vi "Optimize RF Power.vi"(4 "MC Error in":errorcluster, 5 "Lock-in Error In":errorcluster, 6 "Time to read at power [ms]":i32=500, 8 "Spectral Data In":T2={"PDT Amp [v]"=0.0, "RIS Amp [v]"=0.0, "B-Field"=[], "All In-Phase Scan Spectra"=[], "Model Select"=enum."OneCompRISTwoPDT", "Fit Each Scan"=FALSE, "PDT Center [g]"=0.0, "In-Phase Average Spectra"=[], "In-Phase Median Spectra"=[], "Out-Phase Median Spectra"=[], "Out-Phase Average Spectra"=[], "Fit Spectra"=[], "Fit No-Baseline Spectra"=[], "All Out-Phase Scan Spectra"=[], "Baseline Offset Correction"=FALSE, "In-Phase Offset [v]"=0.0, "Out-Phase Offset [v]"=0.0, "Ch2 Input\n(Balance)"=[], "Ch3 Input\n(Phase)"=[], "Ch4 Input\n(AFC)"=[], "Fit Pars"=[], "Fit Pars Errors"=[], "Fit Pars Labels"=[], "Raw Scan DAQ Data"=[], "Bad Scans Indicies"=[], "Good In-Phase Scan Spectra"=[], "Good Out-Phase Scan Spectra"=[], "Bad In-Phase Scan Spectra"=[], "Bad Out-Phase Scan Spectra"=[], "Number of bad scans"=0, "Fit History"=[], "PDT Amp. History/Set [v]"=[], "RIS Amp. History/Set [v]"=[], "RIS Amp. History/Scan [v]"=[], "All Shifted B-Fields"=[], "Good Shifted B-Fields"=[], "Ch5 Input\n(SpO2)"=[], "Ch6 Input\n(BPM)"=[], "Global SNR"=0.0, "Fit Error History"=[], "SNR History"=[]} {"Global SNR" min=0.0; "PDT Center [g]" min=0.0; "RIS Amp [v]" min=0.0; "PDT Amp [v]" min=0.0}, 9 "Hardware Parameters In":T1={"Scan Calibration [G/V]"=0.0, "Modulation Calibration [G/V]"=0.0, "Modulation Phase [deg]"=0.0, "Modulation Frequency [Hz]"=0.0, "Attenuation [dB]"=0, "Input Channel Count"=0, "Time constant"=7, "Sensitivity"=17, "Frequency Output Voltage [V]"=0.0, "Phase Output Voltage [V]"=0.0, "Lock-in Offset Compensation"=FALSE, "RF [GHz]"=0.0, "Q Start"=0.0, "Q End"=0.0, "Balance"=0.0, "Phase Error"=0.0, "AFC Error"=0.0, "AFC"=FALSE, "Magnet Rotation"=FALSE, "Balance Scaling Factor"=1.0, "Phase Error Scaling Factor"=1.0, "AFC Error Scaling Factor"=1.0, "Frequency Counter ID"="", "Sweep Waveform"=enum."Sawtooth", "Q-Factor Scale"=0.0, " Q-Data Scale"=0.0, " Q-Data Offset"=0.0, "Magnet Rotation Slope"=0.0, "Magnet Rotation Offset"=0.0, "Phase Sweep Resolution"=0.0, "Hardware Version Number"="", "Spectrometer ID Number"=0, "Spectrometer Name"="", "Lock in Saturation"=0.0, "Balance Threshold"=0.0, "Phase Error Threshold"=0.0, "AFC Error Threshold"=0.0, "Linear Actuator Length"=0.0, "Lock-in OK?"=FALSE, "Ignore Lock-in Comm. Failure"=FALSE, "Gradient Addresses"=[], "Gradient Calibrations [G/A*mm]"=[], "Gradient Power Supplies"=[], "Lock-in Address"="", "Magnet Type"=enum."RRI", "Camera Names"=[], "Sweep Limit [Gauss]"=0.0, "Modulation Limit [Gauss]"=0.0, "Balance Threshold Exceeded?"=FALSE, "Phase Threshold Exceeded?"=FALSE, "AFC Threshold Exceeded?"=FALSE, "Consecutive Re-tune attempts"=0, "Reverse Sweep Slope [sec]"=0.0, "Reverse Sweep Offset [G]"=0.0, "AFC Field Correction [V/MHz]"=0.0, "Active Gradients (X Y Z)"=[], "SpO2 Calibration [SpO2/V]"=1.0, "Heart Rate Calibration [BPM/V]"=1.0, "Thermocouple Channel"=""} {"Sensitivity" items=["", "2 nV", "5 nV", "10 nV", "20 nV", "50 nV", "100 nV", "200 nV", "500 nV", "1 uV", "2 uV", "5 uV", "10 uV", "20 uV", "50 uV", "100 uV", "200 uV", "500 uV", "1 mV", "2 mV", "5 mV", "10 mV", "20 mV", "50 mV", "100 mV", "200 mV", "500 mV", "1 V"]; "Time constant" items=["10 us", "20 us", "40 us", "80 us", "160 us", "320 us", "640 us", "5 ms", "10 ms", "20 ms", "50 ms", "100 ms", "200 ms", "500 ms", "1 s", "2 s", "5 s", "10 s", "20 s", "50 s", "100 s", "200 s", "500 s", "1 ks", "2 ks", "5 ks", "10 ks", "20 ks", "50 ks", "100 ks"]}) -> (0 "Resultant Attenuation [dB]":u16, 1 "MC error out":errorcluster, 2 "Lock-in error out":errorcluster, 3 "Hardware Parameters Out":T1={"Scan Calibration [G/V]"=0.0, "Modulation Calibration [G/V]"=0.0, "Modulation Phase [deg]"=0.0, "Modulation Frequency [Hz]"=0.0, "Attenuation [dB]"=0, "Input Channel Count"=0, "Time constant"=7, "Sensitivity"=17, "Frequency Output Voltage [V]"=0.0, "Phase Output Voltage [V]"=0.0, "Lock-in Offset Compensation"=FALSE, "RF [GHz]"=0.0, "Q Start"=0.0, "Q End"=0.0, "Balance"=0.0, "Phase Error"=0.0, "AFC Error"=0.0, "AFC"=FALSE, "Magnet Rotation"=FALSE, "Balance Scaling Factor"=1.0, "Phase Error Scaling Factor"=1.0, "AFC Error Scaling Factor"=1.0, "Frequency Counter ID"="", "Sweep Waveform"=enum."Sawtooth", "Q-Factor Scale"=0.0, " Q-Data Scale"=0.0, " Q-Data Offset"=0.0, "Magnet Rotation Slope"=0.0, "Magnet Rotation Offset"=0.0, "Phase Sweep Resolution"=0.0, "Hardware Version Number"="", "Spectrometer ID Number"=0, "Spectrometer Name"="", "Lock in Saturation"=0.0, "Balance Threshold"=0.0, "Phase Error Threshold"=0.0, "AFC Error Threshold"=0.0, "Linear Actuator Length"=0.0, "Lock-in OK?"=FALSE, "Ignore Lock-in Comm. Failure"=FALSE, "Gradient Addresses"=[], "Gradient Calibrations [G/A*mm]"=[], "Gradient Power Supplies"=[], "Lock-in Address"="", "Magnet Type"=enum."RRI", "Camera Names"=[], "Sweep Limit [Gauss]"=0.0, "Modulation Limit [Gauss]"=0.0, "Balance Threshold Exceeded?"=FALSE, "Phase Threshold Exceeded?"=FALSE, "AFC Threshold Exceeded?"=FALSE, "Consecutive Re-tune attempts"=0, "Reverse Sweep Slope [sec]"=0.0, "Reverse Sweep Offset [G]"=0.0, "AFC Field Correction [V/MHz]"=0.0, "Active Gradients (X Y Z)"=[], "SpO2 Calibration [SpO2/V]"=1.0, "Heart Rate Calibration [BPM/V]"=1.0, "Thermocouple Channel"=""} {"Sensitivity" items=["", "2 nV", "5 nV", "10 nV", "20 nV", "50 nV", "100 nV", "200 nV", "500 nV", "1 uV", "2 uV", "5 uV", "10 uV", "20 uV", "50 uV", "100 uV", "200 uV", "500 uV", "1 mV", "2 mV", "5 mV", "10 mV", "20 mV", "50 mV", "100 mV", "200 mV", "500 mV", "1 V"]; "Time constant" items=["10 us", "20 us", "40 us", "80 us", "160 us", "320 us", "640 us", "5 ms", "10 ms", "20 ms", "50 ms", "100 ms", "200 ms", "500 ms", "1 s", "2 s", "5 s", "10 s", "20 s", "50 s", "100 s", "200 s", "500 s", "1 ks", "2 ks", "5 ks", "10 ks", "20 ks", "50 ks", "100 ks"]})   [LabVIEW 2016]
uses:
  Types/Hardware Parameters.ctl
  Types/Spectral Data.ctl
  Types/Fitting Model Selection.ctl
  <vilib>/Analysis/NI_AALBase.lvlib
panel:
  out "Max Attenuation Reached":bool
  out "Live Data at Power":dbl[](graph)
  out "Power Points":dbl[](array[numeric])
  out "Amplitude vs. Attenuation Steps (3db/step)":dbl[](graph)
  out "Optimized Attenuation [dB]":u16 max=31 step=1
  out "Current Attenuation [dB]":u16 max=31 step=1
  in  "Cases":T4(ring)
  # "Bridge I/O"
  # "Magnet Rotation"
  # "Field Calibration"
  # "Lock In Amplifier"
  # "Spectrometer Information"
  # "DAQ Settings"
  # "Gradient Coils and Field"
  # "X"
  # "Y"
  # "Z"
  # "Q-Measurements"
  # "Bridge I/O"
  # "Magnet Rotation"
  # "Field Calibration"
  # "Lock In Amplifier"
  # "Spectrometer Information"
  # "DAQ Settings"
  # "Gradient Coils and Field"
  # "X"
  # "Y"
  # "Z"
  # "Q-Measurements"
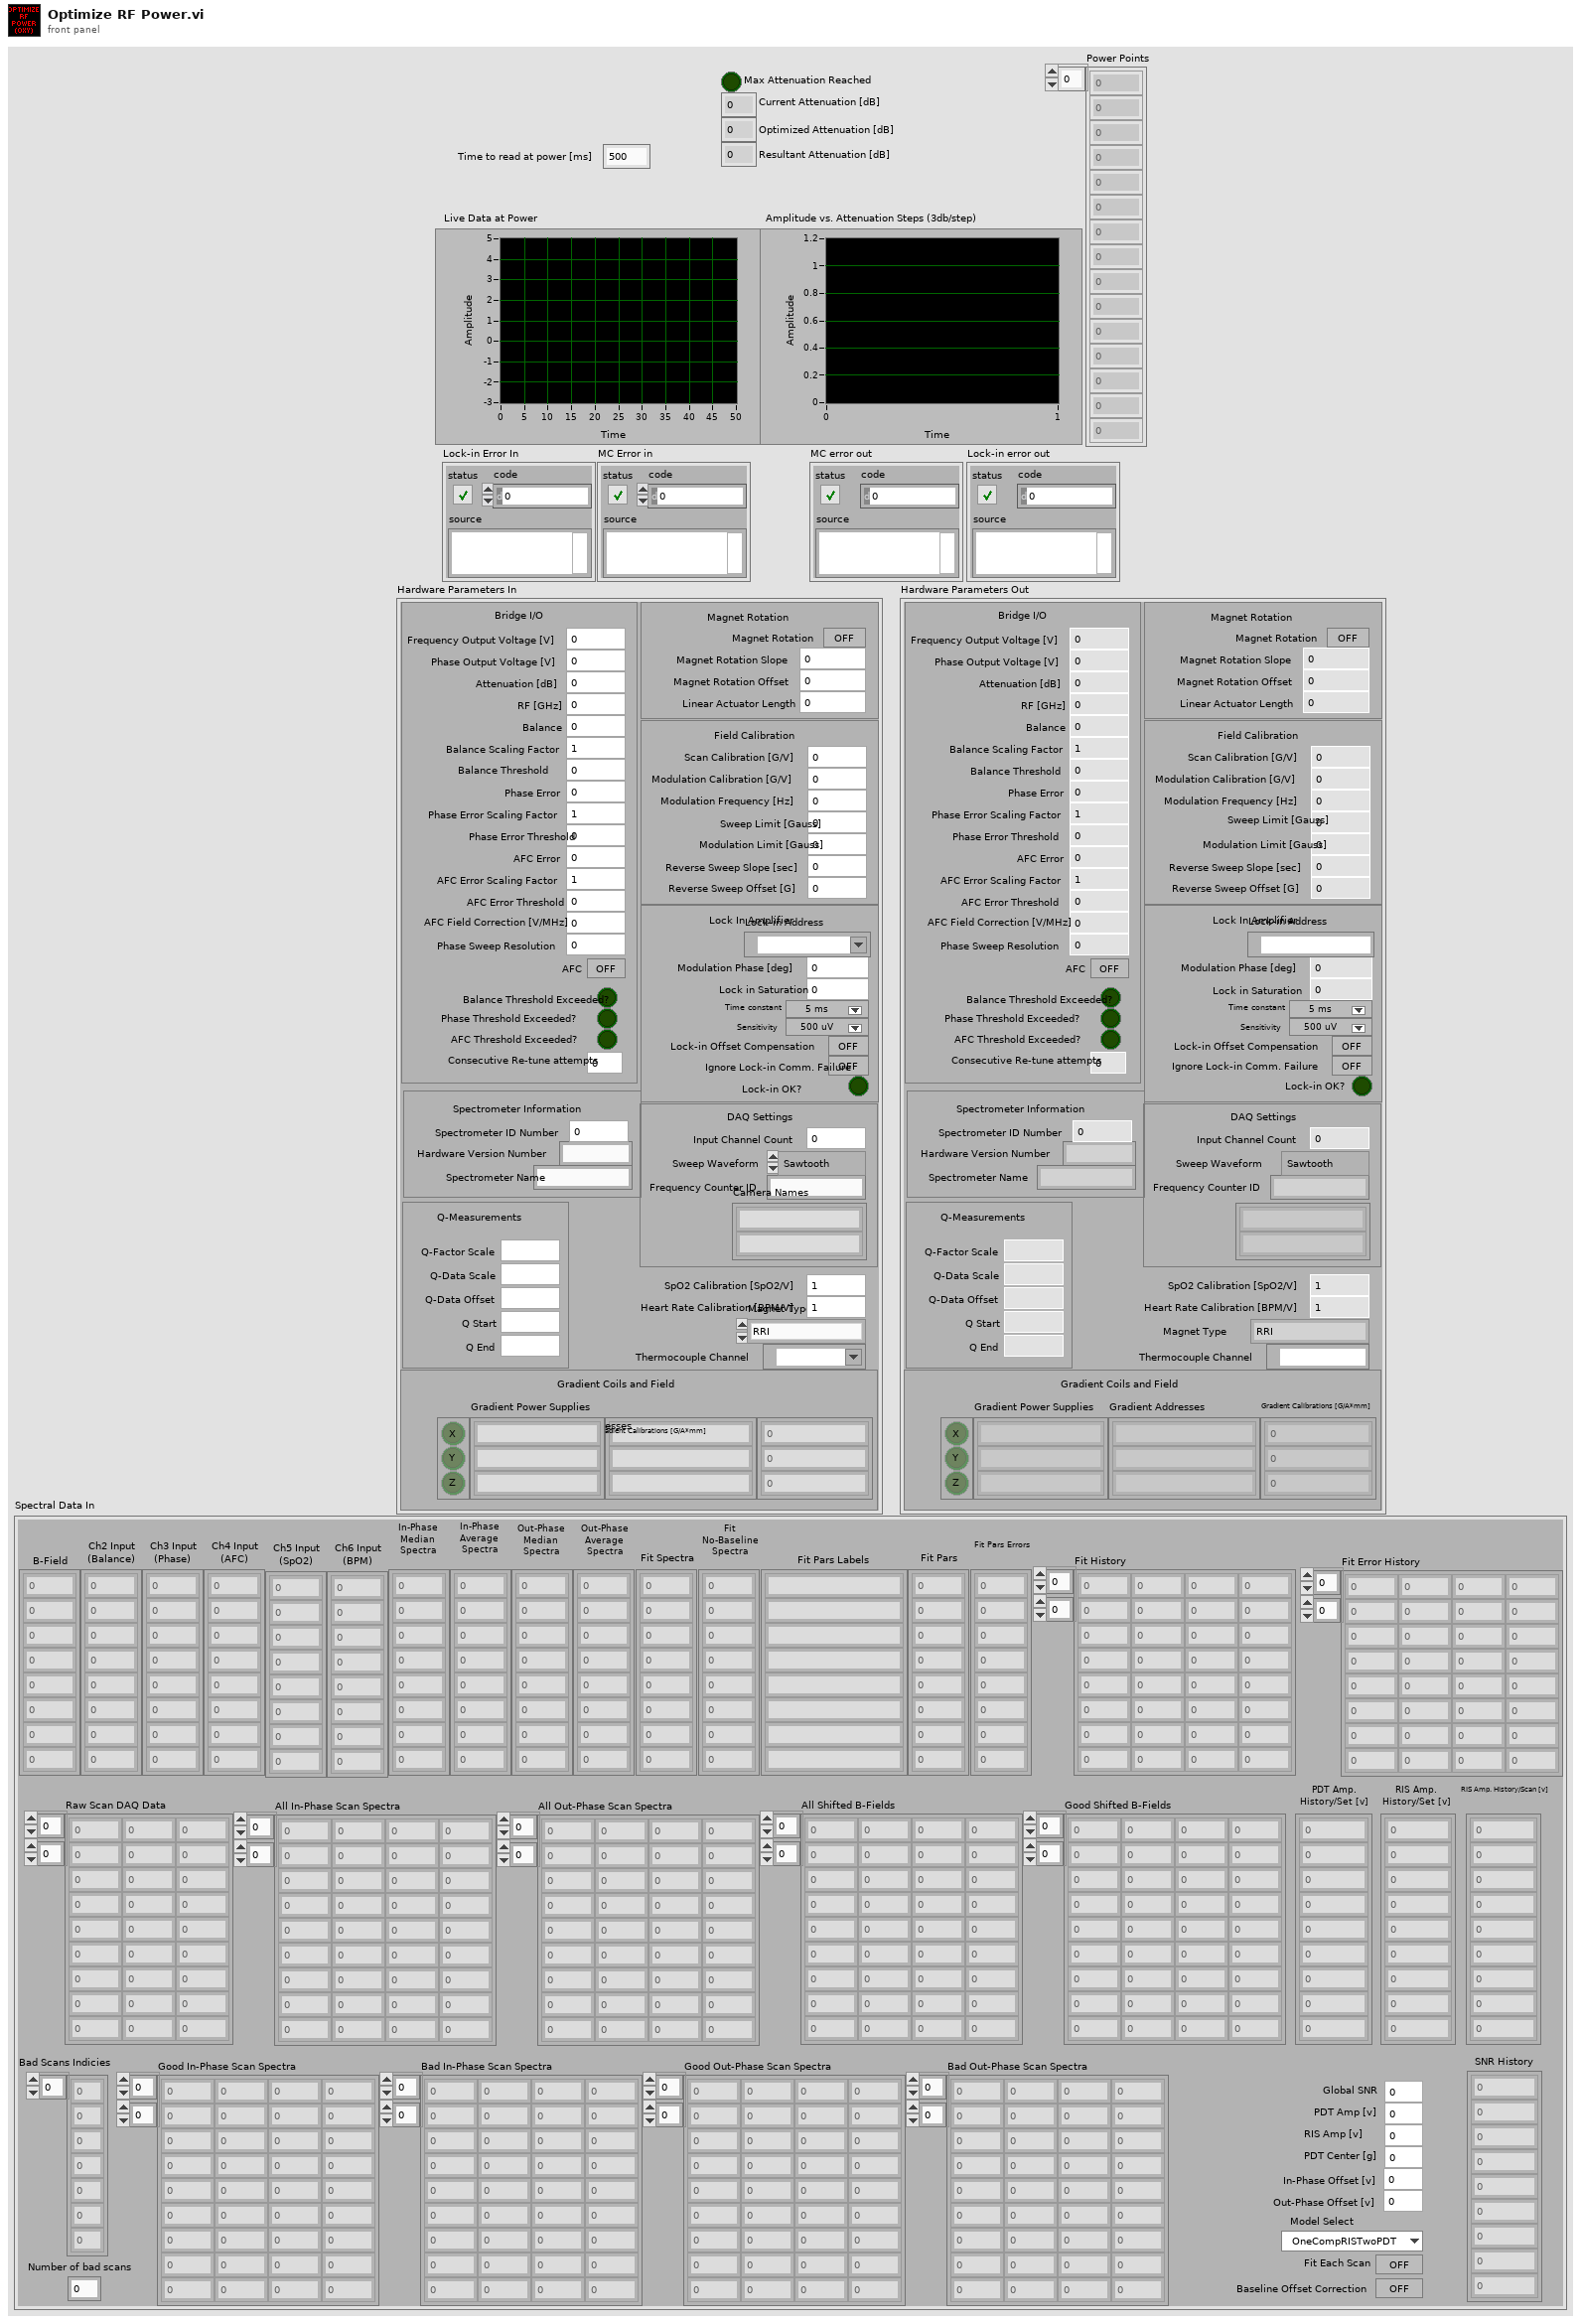
[diagram p1: front panel]
types:
  T1 = typedef "Hardware Parameters.ctl" = cluster{"Scan Calibration [G/V]":dbl, "Modulation Calibration [G/V]":dbl, "Modulation Phase [deg]":dbl, "Modulation Frequency [Hz]":dbl, "Attenuation [dB]":u16, "Input Channel Count":i32, "Time constant":u16, "Sensitivity":u16, "Frequency Output Voltage [V]":dbl, "Phase Output Voltage [V]":dbl, "Lock-in Offset Compensation":bool, "RF [GHz]":dbl, "Q Start":dbl, "Q End":dbl, "Balance":dbl, "Phase Error":dbl, "AFC Error":dbl, "AFC":bool, "Magnet Rotation":bool, "Balance Scaling Factor":dbl, "Phase Error Scaling Factor":dbl, "AFC Error Scaling Factor":dbl, "Frequency Counter ID":string, "Sweep Waveform":enum16{"Sine Wave", "Square Wave", "Sawtooth", "Triangle Wave"}, "Q-Factor Scale":dbl, " Q-Data Scale":dbl, " Q-Data Offset":dbl, "Magnet Rotation Slope":dbl, "Magnet Rotation Offset":dbl, "Phase Sweep Resolution":dbl, "Hardware Version Number":string, "Spectrometer ID Number":i32, "Spectrometer Name":string, "Lock in Saturation":dbl, "Balance Threshold":dbl, "Phase Error Threshold":dbl, "AFC Error Threshold":dbl, "Linear Actuator Length":dbl, "Lock-in OK?":bool, "Ignore Lock-in Comm. Failure":bool, "Gradient Addresses":string[], "Gradient Calibrations [G/A*mm]":dbl[], "Gradient Power Supplies":string[], "Lock-in Address":refnum<visa-resource-name>, "Magnet Type":enum16{"RRI", "BARDA", "Whole Body Permanent", "RRI Electromagnet"}, "Camera Names":string[], "Sweep Limit [Gauss]":dbl, "Modulation Limit [Gauss]":dbl, "Balance Threshold Exceeded?":bool, "Phase Threshold Exceeded?":bool, "AFC Threshold Exceeded?":bool, "Consecutive Re-tune attempts":i32, "Reverse Sweep Slope [sec]":dbl, "Reverse Sweep Offset [G]":dbl, "AFC Field Correction [V/MHz]":dbl, "Active Gradients (X Y Z)":bool[], "SpO2 Calibration [SpO2/V]":dbl, "Heart Rate Calibration [BPM/V]":dbl, "Thermocouple Channel":tag}
  T2 = typedef "Spectral Data.ctl" = cluster{"PDT Amp [v]":dbl, "RIS Amp [v]":dbl, "B-Field":dbl[], "All In-Phase Scan Spectra":dbl[][], "Model Select":T3, "Fit Each Scan":bool, "PDT Center [g]":dbl, "In-Phase Average Spectra":dbl[], "In-Phase Median Spectra":dbl[], "Out-Phase Median Spectra":dbl[], "Out-Phase Average Spectra":dbl[], "Fit Spectra":dbl[], "Fit No-Baseline Spectra":dbl[], "All Out-Phase Scan Spectra":dbl[][], "Baseline Offset Correction":bool, "In-Phase Offset [v]":dbl, "Out-Phase Offset [v]":dbl, "Ch2 Input\n(Balance)":dbl[], "Ch3 Input\n(Phase)":dbl[], "Ch4 Input\n(AFC)":dbl[], "Fit Pars":dbl[], "Fit Pars Errors":dbl[], "Fit Pars Labels":string[], "Raw Scan DAQ Data":dbl[][], "Bad Scans Indicies":i32[], "Good In-Phase Scan Spectra":dbl[][], "Good Out-Phase Scan Spectra":dbl[][], "Bad In-Phase Scan Spectra":dbl[][], "Bad Out-Phase Scan Spectra":dbl[][], "Number of bad scans":i32, "Fit History":dbl[][], "PDT Amp. History/Set [v]":dbl[], "RIS Amp. History/Set [v]":dbl[], "RIS Amp. History/Scan [v]":dbl[], "All Shifted B-Fields":dbl[][], "Good Shifted B-Fields":dbl[][], "Ch5 Input\n(SpO2)":dbl[], "Ch6 Input\n(BPM)":dbl[], "Global SNR":dbl, "Fit Error History":dbl[][], "SNR History":dbl[]}
  T3 = typedef "Fitting Model Selection.ctl" = enum16{"OneCompRIS", "OneCompRISTwoPDT", "OneCompRISRev", "OneCompRISTwoPDTRev", "LiPc", "TwoLiPc", "ThreeLiPc", "FourLiPc", "PDTCalibration", "CE_Ink", "Printex", "MelaninTwoPDT"}
  T4 = enum16{"Delay", "Collect Data", "Reduce Power", "Increase Power", "Compare", "Complete"}
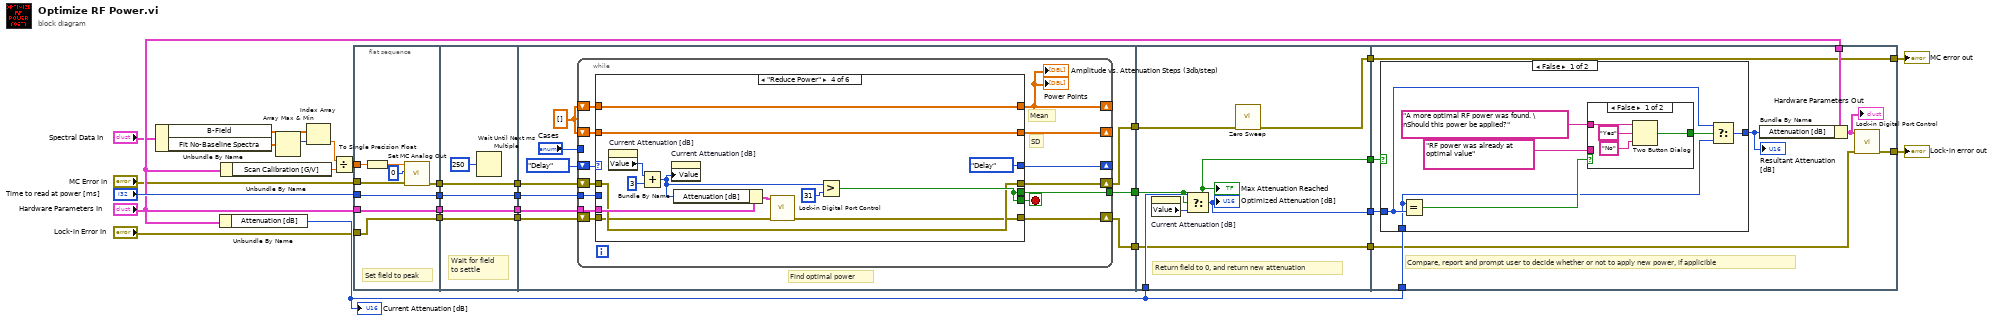
[diagram p0: block diagram]
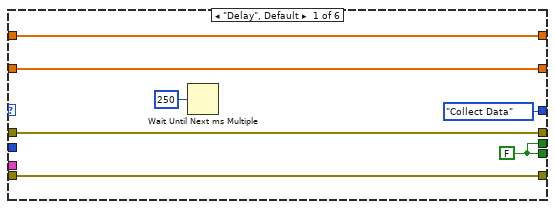
[diagram p2: hidden frame]
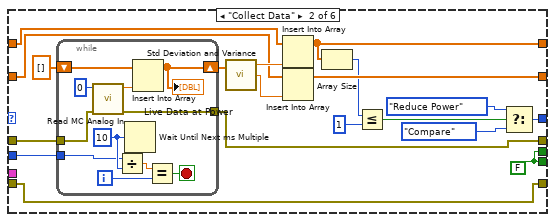
[diagram p3: hidden frame]
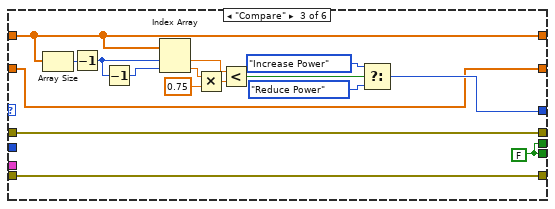
[diagram p4: hidden frame]
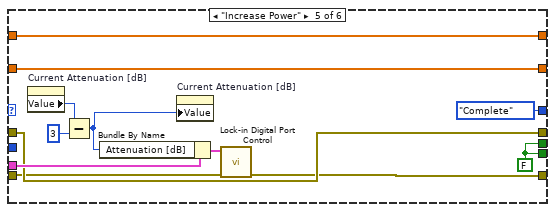
[diagram p5: hidden frame]
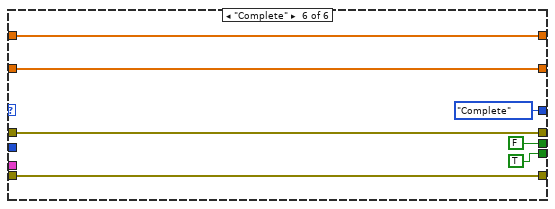
[diagram p6: hidden frame]
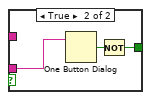
[diagram p7: hidden frame]
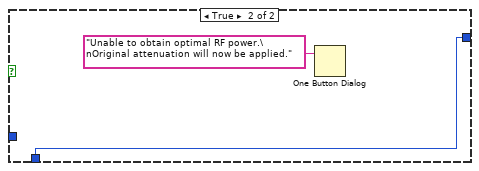
[diagram p8: hidden frame]
diagram:
  n1 = Unbundle By Name("Spectral Data In") -> ("B-Field"=w14:dbl[], "Fit No-Baseline Spectra"=w16:dbl[])
  n2 = Unbundle By Name("Hardware Parameters In") -> ("Attenuation [dB]"=w19:u16)
  "Current Attenuation [dB]" <- w19
  n3 = Unbundle By Name("Hardware Parameters In") -> ("Scan Calibration [G/V]"=w22:dbl)
  n4 = Array Max & Min(array=w16) -> (max index (indices)=w15:i32)  [unwired: 3 out]
  n5 = Index Array(array=w14, index=w15) -> (element=w13:dbl)
  n6 = Divide(x=w13, y=w22) -> (x/y=w29:dbl)
  n7 = flat-sequence {
    tunnel: w29 -> [w35]
    tunnel: "Time to read at power [ms]" -> [w37]
    tunnel: [w37] -> w28
    tunnel: "Hardware Parameters In" -> [w33]
    tunnel: [w33] -> w23
    tunnel: [w32] -> w11
    tunnel: "MC Error in" -> [w31]
    tunnel: "Lock-in Error In" -> [w30]
    tunnel: [w30] -> w7
    tunnel: [w41] -> w27
    tunnel: w28 -> [w41]
    tunnel: [w40] -> w24
    tunnel: w23 -> [w40]
    tunnel: [w39] -> w12
    tunnel: w11 -> [w39]
    tunnel: [w38] -> w8
    tunnel: w7 -> [w38]
    tunnel: w27 -> [w51]
    tunnel: [w48] -> w25
    tunnel: w24 -> [w47]
    tunnel: w12 -> [w46]
    tunnel: w8 -> [w45]
    tunnel: [w44] -> w6
    tunnel: [w43] -> w5
    tunnel: w25 -> [w155]
    tunnel: w19 -> [w158]
    tunnel: [w156] -> w21
    tunnel: [w155] -> w20
    tunnel: w6 -> [w154]
    tunnel: w5 -> [w153]
    tunnel: [w153] -> w4
    tunnel: [w152] -> w3
    tunnel: w21 -> [w167]
    tunnel: w20 -> [w166]
    tunnel: w19 -> [w165]
    tunnel: "Hardware Parameters In" -> [w163]
    tunnel: w4 -> [w161]
    tunnel: w3 -> [w160]
    tunnel: [w160] -> w2
    tunnel: [w159] -> w1
    frame #0 {
      # "Set field to peak"
      n8 = To Single Precision Float(number=w35) -> (single precision float=w34:sgl)
      n9 = call "Set MC Analog Out.vi"("error in (no error)"=w31, "Channel"=0, "Output Voltage"=w34) -> ("error out"=w32:errorcluster)  [unwired: 8 in]
    }
    frame #1 {
      # "Wait for field \nto settle"
      n10 = Wait Until Next ms Multiple(millisecond multiple=u32 250) -> ()  [unwired: 1 out]
    }
    frame #2 {
      w49 = dbl[] []
      # "Find optimal power"
      n11 = while {
        shift-right: [w65] -> _
        shift-left: T4."Delay" ("Cases") -> [w63]
        tunnel: "Cases" -> [_]
        tunnel: w51 -> [w64]
        shift-right: [w59] -> _
        shift-left: w49 -> [w62]
        shift-right: [w61] -> _
        shift-left: w49 -> [w60]
        tunnel: [w58] -> w48
        tunnel: w47 -> [w57]
        shift-right: [w55] -> w44
        shift-left: w46 -> [w56]
        shift-right: [w54] -> w43
        shift-left: w45 -> [w53]
        stop <- w66 stop-if-true
        # "SD"
        # "Mean"
        n12 = case shown="\"Reduce Power\"" w63 {
          tunnel: [w69 w77 w106 w126 w139 TRUE] -> w66
          tunnel: [T4."Collect Data" ("Cases") w80 w119 T4."Delay" ("Cases") T4."Complete" ("Cases") T4."Complete" ("Cases")] -> w65
          tunnel: w64 -> [_ w91 _ _ _ _]
          tunnel: [w71 w85 w115 w130 w142 w149] -> w59
          tunnel: w62 -> [w71 w89 w115 w130 w142 w149]
          tunnel: [w70 w87 w114 w129 w141 w148] -> w61
          tunnel: w60 -> [w70 w86 w114 w129 w141 w148]
          tunnel: [w69 w77 w106 w126 w139 FALSE] -> w58
          tunnel: w57 -> [_ _ _ w125 w136 _]
          tunnel: w56 -> [w68 w76 w105 w122 w135 w146]
          tunnel: [w68 w75 w105 w122 w135 w146] -> w55
          tunnel: [w67 w74 w104 w121 w133 w145] -> w54
          tunnel: w53 -> [w67 w74 w104 w120 w134 w145]
          frame "Delay", Default {
            w69 = FALSE
            n13 = Wait Until Next ms Multiple(millisecond multiple=u32 250) -> ()  [unwired: 1 out]
          }
          frame "Collect Data" {
            w77 = FALSE
            n14 = while {
              shift-right: [w97] -> w92
              shift-left: dbl[] [] -> [w99]
              tunnel: w91 -> [w98]
              tunnel: w76 -> [w94]
              tunnel: [w93] -> w75
              i -> [w103]
              stop <- w102 stop-if-true
              w101 = u32 10 ("millisecond multiple")
              n15 = call "Read MC Analog In.vi"("error in (no error)"=w94, "channel"=0 ("Channel")) -> ("error out"=w93:errorcluster, "Voltage Input"=w96:dbl)  [unwired: 8 in]
              n16 = Divide(x=w98, y=w101) -> (x/y=w100:dbl)
              n17 = Wait Until Next ms Multiple(millisecond multiple=w101) -> ()  [unwired: 1 out]
              n18 = Insert Into Array(array=w99, new element=w96) -> (w97:dbl[])  [unwired: 1 in]
              "Live Data at Power" <- w97
              n19 = Equal?(x=w100, y=w103) -> (x = y?=w102:bool)
            }
            n20 = call <vilib>:"Std Deviation and Variance.vi"("X"=w92) -> ("mean"=w90:dbl, "standard deviation"=w88:dbl)  [unwired: 1 in, 1 out]
            n21 = Insert Into Array(array=w89, new element=w90) -> (w85:dbl[])  [unwired: 1 in]
            n22 = Insert Into Array(array=w86, new element=w88) -> (w87:dbl[])  [unwired: 1 in]
            n23 = Array Size(array=w85) -> (size(s)=w84:i32)
            n24 = Less Or Equal?(x=w84, y=1) -> (x <= y?=w82:bool)
            n25 = Select(t=T4."Reduce Power" ("Cases"), s=w82, f=T4."Compare" ("Cases")) -> (s? t:f=w80:T4)
          }
          frame "Compare" {
            w106 = FALSE
            n26 = Array Size(array=w115) -> (size(s)=w113:i32)
            n27 = Decrement(x=w113) -> (x-1=w111:i32)
            n28 = Decrement(x=w111) -> (x-1=w112:i32)
            n29 = Index Array(array=w115, index #1=w111, index #2=w112) -> (element #1=w108:dbl, element #2=w110:dbl)
            n30 = Multiply(x=w110, y=0.75) -> (x*y=w107:dbl)
            n31 = Less?(x=w108, y=w107) -> (x < y?=w116:bool)
            n32 = Select(t=T4."Increase Power" ("Cases"), s=w116, f=T4."Reduce Power" ("Cases")) -> (s? t:f=w119:T4)
          }
          frame "Reduce Power" {
            n33 = property on="Current Attenuation [dB]" class="DigNum (strict)"() -> ("Value"=w128:u16)  [unwired: 2 in, 2 out]
            n34 = Add(x=w128, y=u16 3) -> (x+y=w123:u16)
            n35 = property on="Current Attenuation [dB]" class="DigNum (strict)"("Value"=w123) -> ()  [unwired: 2 in, 2 out]
            n36 = Bundle By Name(cluster=w125, "Attenuation [dB]"=w123) -> (w124:T1)
            n37 = call "Lock-in Digital Port Control.vi"("error in (no error)"=w120, "Hardware Parameters"=w124) -> ("error out"=w121:errorcluster)  [unwired: 9 in]
            n38 = Greater?(x=w123, y=u16 31) -> (0:w126:bool)
          }
          frame "Increase Power" {
            w139 = FALSE
            n39 = property on="Current Attenuation [dB]" class="DigNum (strict)"() -> ("Value"=w140:u16)  [unwired: 2 in, 2 out]
            n40 = Subtract(x=w140, y=u16 3) -> (x-y=w137:u16)
            n41 = Bundle By Name(cluster=w136, "Attenuation [dB]"=w137) -> (w138:T1)
            n42 = property on="Current Attenuation [dB]" class="DigNum (strict)"("Value"=w137) -> ()  [unwired: 2 in, 2 out]
            n43 = call "Lock-in Digital Port Control.vi"("error in (no error)"=w134, "Hardware Parameters"=w138) -> ("error out"=w133:errorcluster)  [unwired: 9 in]
          }
          frame "Complete" {
          }
        }
        "Amplitude vs. Attenuation Steps (3db/step)" <- w59
        "Power Points" <- w59
      }
    }
    frame #3 {
      # "Return field to 0, and return new attenuation"
      n44 = property on="Current Attenuation [dB]" class="DigNum (strict)"() -> ("Value"=w157:u16)  [unwired: 2 in, 2 out]
      n45 = Select(t=w158, s=w155, f=w157) -> (s? t:f=w156:u16)
      "Optimized Attenuation [dB]" <- w156
      n46 = call "Zero Sweep.vi"("error in (no error)"=w154) -> ("error out"=w152:errorcluster)  [unwired: 10 in]
      "Max Attenuation Reached" <- w155
    }
    frame #4 {
      # "Compare, report and prompt user to decide whether or not to apply new power, if applicible"
      n47 = case shown="False" w166 {
        tunnel: w167 -> [w170 _]
        tunnel: w165 -> [w169 w182]
        tunnel: [w168 w182] -> w164
        frame False {
          n48 = Equal?(x=w169, y=w170) -> (x = y?=w172:bool)
          n49 = case shown="False" w172 {
            tunnel: "RF power was already at optimal value" ("message") -> [_ w181]
            tunnel: "A more optimal RF power was found. \nShould this power be applied?" ("message") -> [w176 _]
            tunnel: [w175 w179] -> w171
            frame False {
              n50 = Two Button Dialog(message=w176, 1:"No" ("F button name (\"Cancel\")"), 2:"Yes" ("T button name (\"OK\")")) -> (T button?=w175:bool)
            }
            frame True {
              n51 = One Button Dialog(message=w181) -> (true=w180:bool)  [unwired: 1 in]
              n52 = Not(x=w180) -> (.not. x?=w179:bool)
            }
          }
          n53 = Select(t=w170, s=w171, f=w169) -> (s? t:f=w168:u16)
        }
        frame True {
          n54 = One Button Dialog(message="Unable to obtain optimal RF power.\nOriginal attenuation will now be applied.") -> ()  [unwired: 1 in, 1 out]
        }
      }
      "Resultant Attenuation [dB]" <- w164
      n55 = Bundle By Name(cluster=w163, "Attenuation [dB]"=w164) -> (w162:T1)
      "Hardware Parameters Out" <- w162
      n56 = call "Lock-in Digital Port Control.vi"("error in (no error)"=w161, "Hardware Parameters"=w162) -> ("error out"=w159:errorcluster)  [unwired: 9 in]
    }
  }
  "MC error out" <- w2
  "Lock-in error out" <- w1
